vi "Read Buffer.vi"(8 "error in":errorcluster, 9 "timeout ms (0)":i32 format="%d ms", 10 "byte order (little-endian)":T1=enum."little-endian", 11 "queue data in":T2={"server ID"=refnum, "Buffer data"={"decimation"=0, "avg bandwidth"=0.0, "channels"=[], "byte order"=enum."little-endian", "buffer descriptor"={"buffer type"=enum."Engine", "plugin id"=0, "group id"=0, "transfer id"=0, "offset"=0, "length"=0}, "values channels"={"index"=0, "count"=0, "engine offset"=0}, "select start offset"=18446744073709551615, "select end offset"=0, "channel index"=-1}} {"Buffer data"."channels"."configuration"."string offset" format="%d bytes"; "Buffer data"."avg bandwidth" format="%.0g bytes"}) -> (0 "error out":errorcluster, 1 "buffer data":string, 2 "values string":string, 3 "queue data out":T2={"server ID"=refnum, "Buffer data"={"decimation"=0, "avg bandwidth"=0.0, "channels"=[], "byte order"=enum."little-endian", "buffer descriptor"={"buffer type"=enum."Engine", "plugin id"=0, "group id"=0, "transfer id"=0, "offset"=0, "length"=0}, "values channels"={"index"=0, "count"=0, "engine offset"=0}, "select start offset"=18446744073709551615, "select end offset"=0, "channel index"=-1}} {"Buffer data"."channels"."configuration"."string offset" format="%d bytes"; "Buffer data"."avg bandwidth" format="%.0g bytes"}, 4 "timed out?":bool, 5 "buffer size":u64, 7 "metrics":T11)   [LabVIEW 2020, in "DSF Core.lvlib"]
uses:
  DSF Core.lvlib
  Typedefs/DSF Data Type.ctl
  Buffer Data.ctl
  Typedefs/DSF Settings Info.ctl
  Typedefs/DSF Byte Order.ctl
  Typedefs/DSF Buffer Type.ctl
  Classes/Thread/Data Server/DSF Buffer Subset Descriptor.ctl
  Queue Data.ctl
  Classes/Thread/Data Server/Metrics.ctl
  Classes/Thread/Data Server/Data Server Thread.lvclass
  Main VI/Values Channels.ctl
  Typedefs/Core Channel Configuration.ctl
  Classes/Configuration/Core/Channel/Channel Configuration.lvclass
  Classes/Configuration/Core/Transfer/Channel Configuration.ctl
  Classes/Configuration/Core/Transfer/Transfer Configuration.lvclass
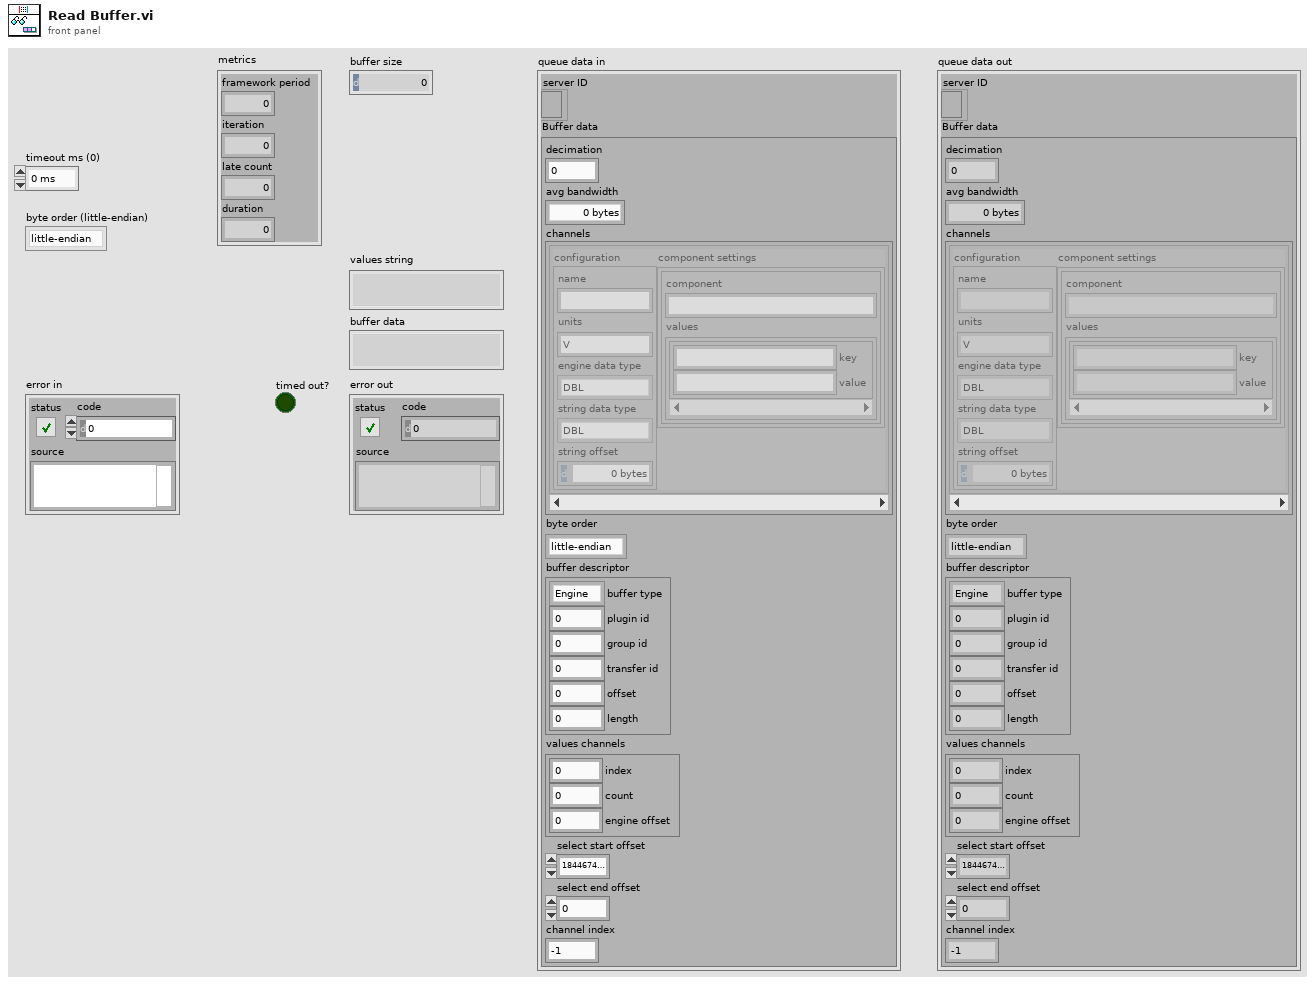
[diagram p1: front panel]
types:
  T1 = typedef "DSF Core.lvlib/DSF Byte Order.ctl" = enum8{"big-endian", "little-endian"}
  T2 = typedef "DSF Core.lvlib/Queue Data.ctl" = cluster{"server ID":refnum<k5>, "Buffer data":T3}
  T3 = typedef "DSF Core.lvlib/Buffer Data.ctl" = cluster{"decimation":u64, "avg bandwidth":dbl, "channels":T4[], "byte order":T1, "buffer descriptor":T8, "values channels":T10, "select start offset":u64, "select end offset":u64, "channel index":i32}
  T4 = typedef "DSF Core.lvlib/Transfer Configuration.lvclass/Channel Configuration.ctl" = cluster{"configuration":T5, "component settings":T7[]}
  T5 = typedef "DSF Core.lvlib/Channel Configuration.lvclass/Core Channel Configuration.ctl" = cluster{"name":string, "units":string, "engine data type":T6, "string data type":T6, "string offset":u64}
  T6 = typedef "DSF Core.lvlib/DSF Data Type.ctl" = enum8{"Bool", "SGL", "DBL", "I8", "I16", "I32", "I64", "U8", "U16", "U32", "U64"}
  T7 = typedef "DSF Core.lvlib/DSF Settings Info.ctl" = cluster{"component":string, "values":cluster{"key":string, "value":string}[]}
  T8 = typedef "DSF Core.lvlib/DSF Buffer Subset Descriptor.ctl" = cluster{"buffer type":T9, "plugin id":i32, "group id":i32, "transfer id":i32, "offset":u64, "length":i64}
  T9 = typedef "DSF Core.lvlib/DSF Buffer Type.ctl" = enum16{"Engine", "String"}
  T10 = typedef "DSF Core.lvlib/Values Channels.ctl" = cluster{"index":i32, "count":i32, "engine offset":u64}
  T11 = typedef "DSF Core.lvlib/Data Server Thread.lvclass/Metrics.ctl" = cluster{"framework period":u32, "iteration":u64, "late count":u64, "duration":u64}
  T12 = cluster{"buffer type":bool, "plugin id":bool, "group id":bool, "transfer id":bool, "offset":bool, "length":bool}
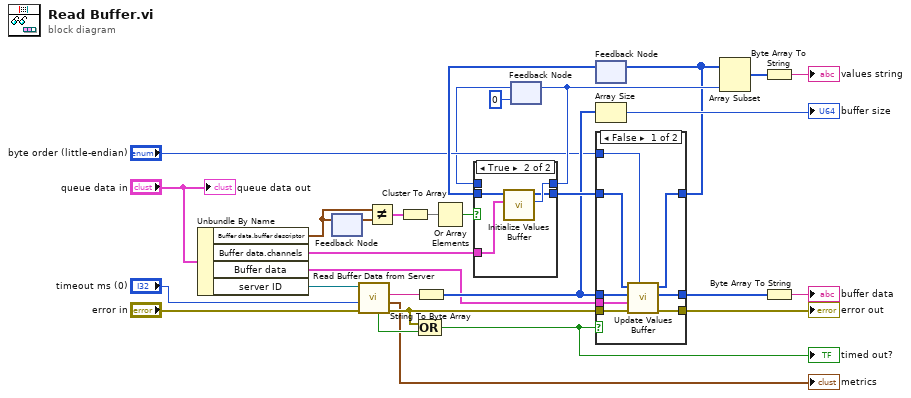
[diagram p0: block diagram]
diagram:
  n1 = Unbundle By Name("queue data in") -> ("Buffer data.buffer descriptor"=w1:T8, "Buffer data.channels"=w2:T4[], "Buffer data"=w10:T3, "server ID"=w28:refnum<k5>)
  n2 = feedback-in #1(w1) -> ()
  n3 = feedback #1() -> (w9:T8)  [unwired: 1 in]
  n4 = call "Read Buffer Data from Server.vi"("error in (no error)"="error in", "timeout ms (25000)"="timeout ms (0)", "server ID in"=w28) -> ("error out"=w23:errorcluster, "metrics"=→"metrics":T11, "buffer data"=w26:string, "timed out?"=w24:bool)  [unwired: 4 in, 1 out]
  n5 = Not Equal?(x=w1, y=w9) -> (x != y?=w8:T12)
  n6 = Cluster To Array(cluster=w8) -> (array=w7:bool[])
  n7 = String To Byte Array(string=w26) -> (unsigned byte array=w15:u8[])
  n8 = Compound Arithmetic op=OR(w23, w24) -> (w14:bool)
  "timed out?" <- w14
  n9 = Or Array Elements(Boolean array=w7) -> (logical OR=w3:bool)
  n10 = feedback #2(0 ("size")) -> (w4:i32)
  n11 = feedback #3() -> (w19:u8[])  [unwired: 1 in]
  n12 = case shown="True" w3 {
    tunnel: [w32 w33] -> w20
    tunnel: w19 -> [w32 w34]
    tunnel: [w31 w36] -> w13
    tunnel: w4 -> [w31 _]
    tunnel: w2 -> [_ w35]
    frame False {
    }
    frame True {
      n13 = call "Initialize Values Buffer.vi"("channels"=w35, "values buffer in"=w34) -> ("size"=w36:i32, "values buffer out"=w33:u8[])  [unwired: 8 in]
    }
  }
  n14 = feedback-in #2(w13) -> ()
  n15 = Array Size(array=w15) -> (size(s)=→"buffer size":i32)
  n16 = case shown="False" w14 {
    tunnel: [w42 w46] -> w30
    tunnel: [w38 _] -> w11
    tunnel: w10 -> [w41 _]
    tunnel: w23 -> [w44 w46]
    tunnel: w15 -> [w43 _]
    tunnel: w20 -> [w39 w45]
    tunnel: [w40 w45] -> w6
    tunnel: "byte order (little-endian)" -> [w37 _]
    frame False {
      n17 = call "Update Values Buffer.vi"("byte order (little-endian)"=w37, "error in"=w44, "buffer data"=w41, "buffer in"=w43, "values buffer in"=w39) -> ("error out"=w42:errorcluster, "buffer out"=w38:u8[], "values buffer out"=w40:u8[])  [unwired: 4 in]
    }
    frame True {
    }
  }
  "error out" <- w30
  n18 = feedback-in #3(w6) -> ()
  n19 = Array Subset(array=w6, length=w13) -> (w18:u8[])  [unwired: 1 in]
  n20 = Byte Array To String(unsigned byte array=w18) -> (string=→"values string":string)
  n21 = Byte Array To String(unsigned byte array=w11) -> (string=→"buffer data":string)
  "queue data out" <- "queue data in"
